vi "Get Multiline Strin.vi"(8 "error in":errorcluster, 11 "Serial Session in":refnum<class "Serial Session.lvclass">) -> (0 "error out":errorcluster, 2 "Data Out":string, 3 "Serial Session out":refnum<class "Serial Session.lvclass">)   [LabVIEW 2016, in "Serial Session.lvclass"]
doc: "In instances where we expect a multiple line string with termination enabled, we don't want to loop through the read calls while dropping the reference with each read. This VI retains the reference while attempting to read and will read until no more characters are returned. Each line will be dumped into an array which can be parsed by the caller."
uses:
  Serial Session.lvclass
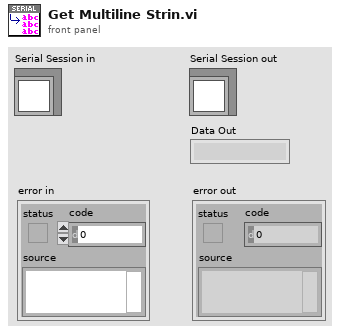
[diagram p1: front panel]
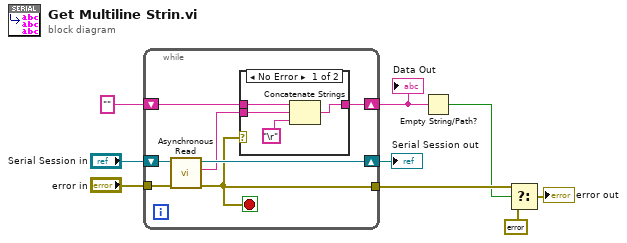
[diagram p0: block diagram]
diagram:
  n1 = while {
    shift-right: [w14] -> w4
    shift-left: "Serial Session in" -> [w16]
    shift-right: [w11] -> w2
    shift-left: "" -> [w15]
    tunnel: "error in" -> [w12]
    tunnel: [w10] -> w7
    stop <- w10 stop-if-true
    n2 = call-dynamic "Asynchronous Read.vi"("error in"=w12, "Serial Session in"=w16) -> ("error out"=w10:errorcluster, "Data Out"=w13:string, "Serial Session out"=w14:refnum<class "Serial Session.lvclass">)  [unwired: 7 in]
    n3 = case shown="No Error" w10 {
      tunnel: w15 -> [w20 w21]
      tunnel: w13 -> [w19 _]
      tunnel: [w18 w21] -> w11
      frame No Error {
        n4 = Concatenate Strings(w20, w19, "\r") -> (w18:string)
      }
      frame Error {
      }
    }
  }
  "Serial Session out" <- w4
  "Data Out" <- w2
  n5 = Empty String/Path?(string/path=w2) -> (empty?=w1:bool)
  n6 = Select(t=w7, s=w1, f=errorcluster {"status"=FALSE, "code"=0, "source"=""} ("error out")) -> (s? t:f=→"error out":errorcluster)
